vi "DAQ Close.vi"(8 "error in (no error)":errorcluster, 11 "DAQ Task":refnum<k21>) -> (0 "error out":errorcluster)   [LabVIEW 2022 SP3]
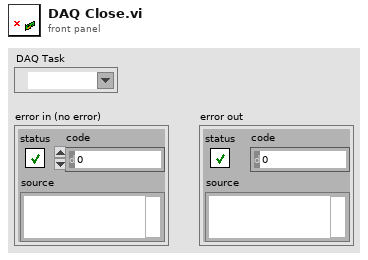
[diagram p1: front panel]
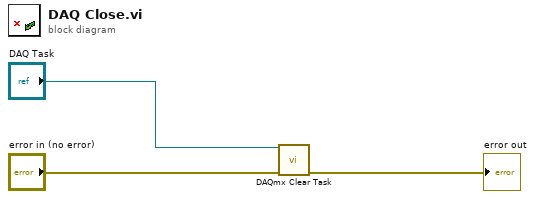
[diagram p0: block diagram]
diagram:
  n1 = call <vilib>:"DAQmx Clear Task.vi"("task in"="DAQ Task", "error in"="error in (no error)") -> ("error out"=→"error out":errorcluster)  [unwired: 13 in]
